vi "Cryostation Client.vi"(8 "error in (no error)":errorcluster, 9 "Data":variant, 10 "Command":T1, 11 "instrument.Cryostation in":refnum<class "instrument.Cryostation.lvclass">) -> (0 "error out":errorcluster, 1 "Data out":variant, 2 "Command out":string, 3 "instrument.Cryostation out":refnum<class "instrument.Cryostation.lvclass">)   [LabVIEW 2016, in "instrument.Cryostation.lvclass"]
uses:
  instrument.Cryostation.lvclass
  C:/Program Files (x86)/National Instruments/LabVIEW 2016/user.lib/LevyLab/Levylab Instruments/SMOs/Instrument/Instrument.lvclass
  Typedefs/Commands-enum.ctl
  <userlib>/LevyLab/Levylab Instruments/SMOs/Instrument/Typedefs/SMO Configuration--Cluster.ctl
  <userlib>/LevyLab/Levylab Instruments/SMOs/Instrument/Typedefs/SMO RC Type--enum.ctl
  <userlib>/LevyLab/Levylab Instruments/SMOs/Instrument/Instrument.lvclass/Instrument.ctl
  <userlib>/LevyLab/Levylab Instruments/SMOs/Instrument/Instrument.lvclass
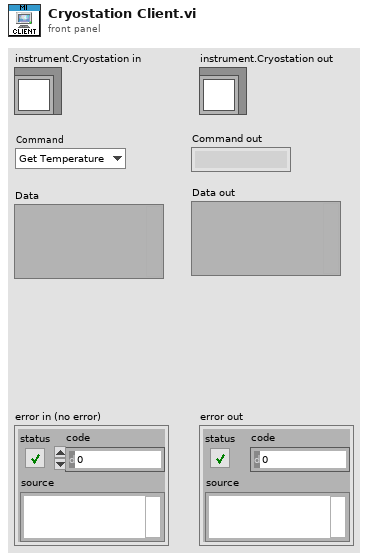
[diagram p1: front panel]
types:
  T1 = typedef "instrument.Cryostation.lvclass/Commands-enum.ctl" = enum16{"Get Temperature", "getAll"}
  T2 = typedef "Instrument.lvclass/SMO RC Type--enum.ctl" = enum16{"RC", "STM", "ZMQ"}
  T3 = typedef "Instrument.lvclass/SMO Configuration--Cluster.ctl" = cluster{"Address":string, "Port":u16, "RC Type":T2}
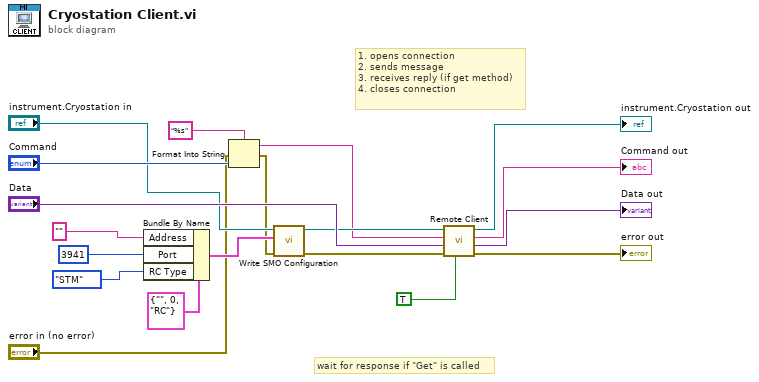
[diagram p0: block diagram]
diagram:
  # "1. opens connection\n2. sends message\n3. receives reply (if get method)\n4. closes connection"
  # "wait for response if \"Get\" is called"
  n1 = Bundle By Name(cluster=T3 {"Address"="", "Port"=0, "RC Type"=enum."RC"} ("SMO"), "Address"="", "Port"=u16 3941, "RC Type"=SMO_RC_Type--enum."STM") -> (w7:T3)
  n2 = Format Into String(format string="%s", error in="error in (no error)", "Command") -> (resulting string=w1:string, error out=w2:errorcluster)  [unwired: 1 in]
  n3 = call <userlib>:"Write SMO Configuration.vi"("error in (no error)"=w2, "SMO"=w7, "Instrument in"="instrument.Cryostation in") -> ("error out"=w12:errorcluster, "Instrument out"=w13:refnum<class "instrument.Cryostation.lvclass">)  [unwired: 7 in]
  n4 = call-dynamic "Remote Client.vi"("Wait for Response?"=TRUE, "error in (no error)"=w12, "Data"="Data", "Command"=w1, "Instrument in"=w13) -> ("error out"=→"error out":errorcluster, "Data out"=→"Data out":variant, "Command out"=→"Command out":string, "Instrument out"=→"instrument.Cryostation out":refnum<class "instrument.Cryostation.lvclass">)  [unwired: 3 in]
